vi "Total costs of all papers.vi"(4 "Instances in":T2[](array[typedef]), 5 "Month days in":timestamp[](array[timestamp]), 6 "error in (no error)":errorcluster, 9 "Refnum in":T1) -> (0 "error out":errorcluster, 1 "Total costs":dbl[](array[numeric]), 3 "Refnum out":T1)   [LabVIEW 2015]
uses:
  Home/Undelivered instance.ctl
  <vilib>/Utility/config.llb/Config Data RefNum.ctl
  <vilib>/Utility/config.llb/NI_LVConfig.lvlib
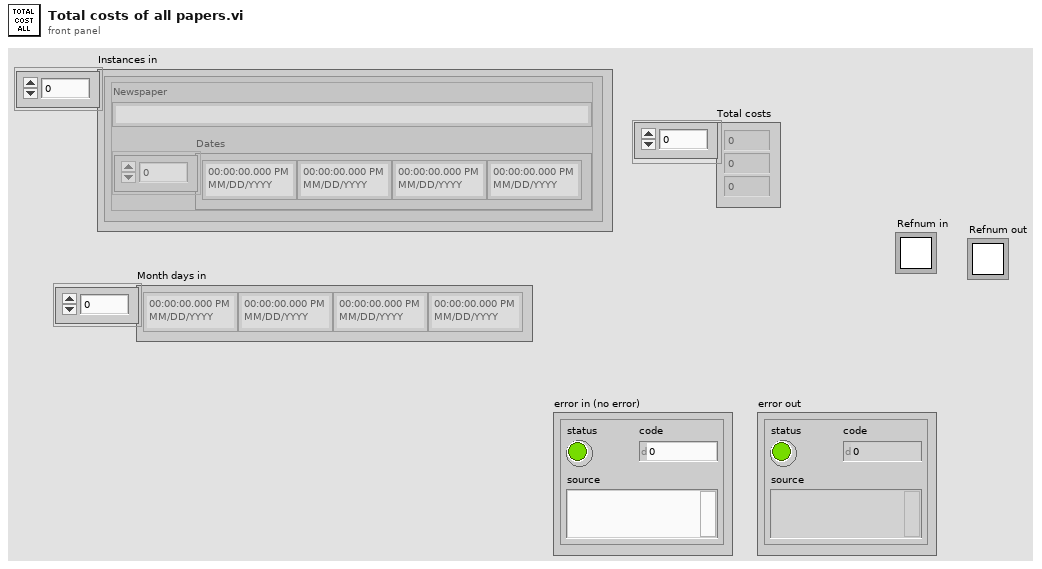
[diagram p1: front panel]
types:
  T1 = typedef "NI_LVConfig.lvlib/Config Data RefNum.ctl" = refnum<k1>
  T2 = typedef "Undelivered instance.ctl" = cluster{"Dates":timestamp[], "Newspaper":string}
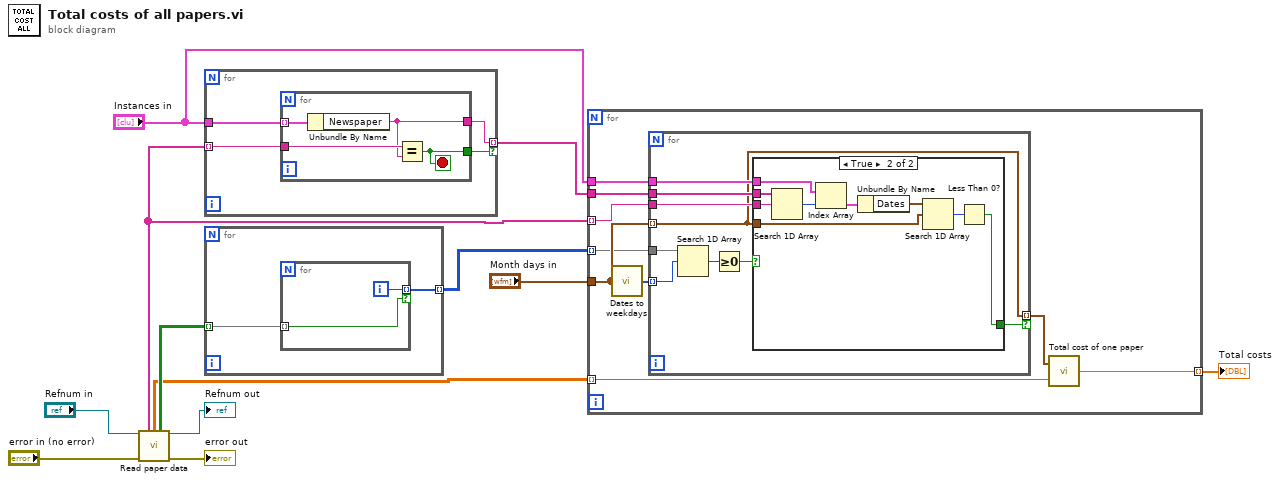
[diagram p0: block diagram]
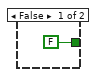
[diagram p2: hidden frame]
diagram:
  n1 = call "Read paper data.vi"("Refnum in"="Refnum in", "error in (no error)"="error in (no error)") -> ("Names"=w10:string[], "Costs"=w6:dbl[][], "Days"=w12:bool[][], "Refnum out"=→"Refnum out":T1, "error out"=→"error out":errorcluster)  [unwired: 9 in]
  n2 = for {
    tunnel: w10 -> [w15] mode=indexing
    tunnel: "Instances in" -> [w16]
    tunnel: [w14] -> w7 mode=indexing if=w13
    n3 = for {
      tunnel: w16 -> [w20] mode=indexing
      tunnel: w15 -> [w19]
      tunnel: [w17] -> w14
      tunnel: [w18] -> w13
      stop <- w18 stop-if-true
      n4 = Unbundle By Name(w20) -> ("Newspaper"=w17:string)
      n5 = Equal?(x=w19, y=w17) -> (x = y?=w18:bool)
    }
  }
  n6 = for {
    tunnel: w12 -> [w22] mode=indexing
    tunnel: [w21] -> w9 mode=indexing
    n7 = for {
      tunnel: w22 -> [w23] mode=indexing
      tunnel: [w24] -> w21 mode=indexing if=w23
      i -> [w24]
    }
  }
  n8 = for {
    tunnel: "Month days in" -> [w33]
    tunnel: w10 -> [w28] mode=indexing
    tunnel: w9 -> [w31] mode=indexing
    tunnel: "Instances in" -> [w30]
    tunnel: w7 -> [w29]
    tunnel: w6 -> [w27] mode=indexing
    tunnel: [w25] -> w5 mode=indexing
    n9 = call "Dates to weekdays.vi"("Dates"=w33) -> ("Weekdays"=w32:i32[])
    n10 = for {
      tunnel: w33 -> [w35] mode=indexing
      tunnel: w32 -> [w36] mode=indexing
      tunnel: w31 -> [w42]
      tunnel: w30 -> [w39]
      tunnel: w29 -> [w38]
      tunnel: w28 -> [w37]
      tunnel: [w35] -> w26 mode=indexing if=w34
      n11 = Search 1D Array(1D array=w42, element=w36) -> (index of element=w41:i32)  [unwired: 1 in]
      n12 = Greater Or Equal To 0?(x=w41) -> (x >= 0?=w40:bool)
      n13 = case shown="True" w40 {
        tunnel: w35 -> [_ w46]
        tunnel: w39 -> [_ w52]
        tunnel: w38 -> [_ w51]
        tunnel: w37 -> [_ w50]
        tunnel: [FALSE w44] -> w34
        frame False {
        }
        frame True {
          n14 = Search 1D Array(1D array=w51, element=w50) -> (index of element=w49:i32)  [unwired: 1 in]
          n15 = Index Array(array=w52, index=w49) -> (element=w48:T2)
          n16 = Unbundle By Name(w48) -> ("Dates"=w47:timestamp[])
          n17 = Search 1D Array(1D array=w47, element=w46) -> (index of element=w45:i32)  [unwired: 1 in]
          n18 = Less Than 0?(x=w45) -> (x < 0?=w44:bool)
        }
      }
    }
    n19 = call "Total cost of one paper.vi"("Cost per day"=w27, "Dates received"=w26) -> ("Total cost"=w25:dbl)
  }
  "Total costs" <- w5
